vi "inteference V3.vi"(7 "number of points":i32, 8 "complex region":T1={"max re"=5.161869466666667e-06, "min re"=5.176843333333334e-06, "max im"=-2.467216e-05, "min im"=-0.001573233, "delta re"=0.003211203, "delta im"=0.00165815, "center re"=0.0015485608400000002, "delta  z"=0.0015530530000000002+0.0i, "center im"=0.0, "center z"=0.0+0.0i, "d im"=0.0, "d re"=0.0, "d z"=0.0+0.0i}, 9 "pond":cdb[][](array[numeric]), 10 "point sources":cdb[](array[numeric]), 11 "wave packet":cdb[][](array[numeric])) -> (3 "pond out":cdb[][](array[numeric]))   [LabVIEW 2010]
uses:
  complex region.ctl
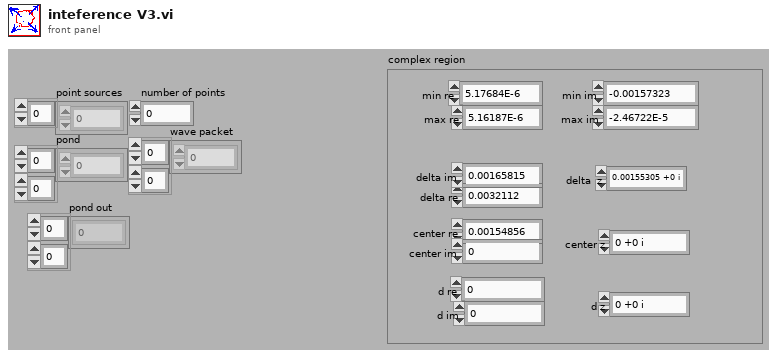
[diagram p1: front panel]
types:
  T1 = typedef "complex region.ctl" = cluster{"max re":dbl, "min re":dbl, "max im":dbl, "min im":dbl, "delta re":dbl, "delta im":dbl, "center re":dbl, "delta  z":cdb, "center im":dbl, "center z":cdb, "d im":dbl, "d re":dbl, "d z":cdb}
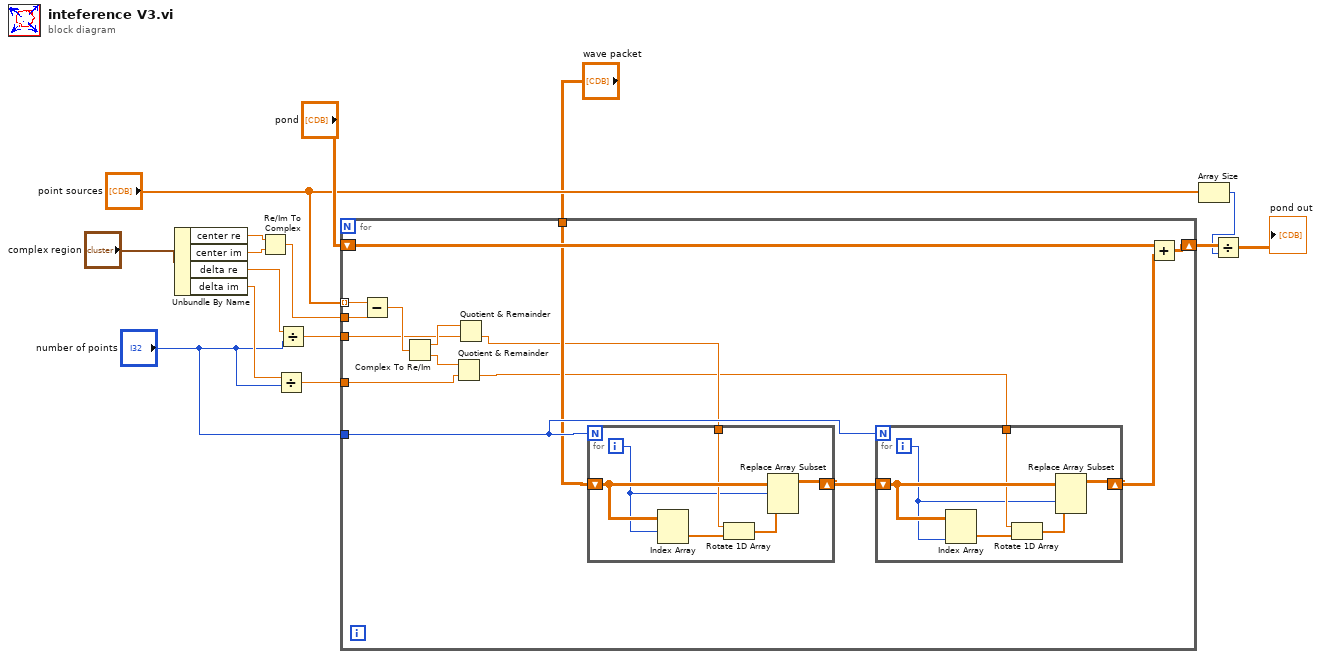
[diagram p0: block diagram]
diagram:
  n1 = Unbundle By Name("complex region") -> ("center re"=w15:dbl, "center im"=w14:dbl, "delta re"=w5:dbl, "delta im"=w4:dbl)
  n2 = Re/Im To Complex(1:w14, 2:w15) -> (0:w13:cdb)
  n3 = Divide(x=w4, y="number of points") -> (x/y=w2:dbl)
  n4 = Divide(x=w5, y="number of points") -> (x/y=w3:dbl)
  n5 = for {
    shift-right: [w29] -> w12
    shift-left: "pond" -> [w30]
    tunnel: "point sources" -> [w28] mode=indexing
    tunnel: "wave packet" -> [w18]
    tunnel: w13 -> [w27]
    tunnel: w3 -> [w24]
    tunnel: w2 -> [w22]
    tunnel: "number of points" -> [w20]
    n6 = Subtract(x=w28, y=w27) -> (x-y=w26:cdb)
    n7 = Complex To Re/Im(x + iy=w26) -> (x=w25:dbl, y=w23:dbl)
    n8 = Quotient & Remainder(x=w23, y=w22) -> (floor(x/y)=w16:dbl)  [unwired: 1 out]
    n9 = Quotient & Remainder(x=w25, y=w24) -> (floor(x/y)=w17:dbl)  [unwired: 1 out]
    n10 = for {
      N: w20 -> [_]
      shift-right: [w42] -> w21
      shift-left: w18 -> [w41]
      tunnel: w17 -> [w38]
      i -> [w37]
      n11 = Index Array(array=w41, index (row)=w37) -> (element=w39:cdb[])  [unwired: 1 in]
      n12 = Rotate 1D Array(1:w39, 2:w38) -> (0:w40:cdb[])
      n13 = Replace Array Subset(array=w41, new element=w40, index (row)=w37) -> (w42:cdb[][])  [unwired: 1 in]
    }
    n14 = for {
      N: w20 -> [_]
      shift-right: [w36] -> w19
      shift-left: w21 -> [w35]
      tunnel: w16 -> [w32]
      i -> [w31]
      n15 = Index Array(array=w35, index (col)=w31) -> (element=w33:cdb[])  [unwired: 1 in]
      n16 = Rotate 1D Array(1:w33, 2:w32) -> (0:w34:cdb[])
      n17 = Replace Array Subset(array=w35, new element=w34, index (col)=w31) -> (w36:cdb[][])  [unwired: 1 in]
    }
    n18 = Add(x=w30, y=w19) -> (x+y=w29:cdb[][])
  }
  n19 = Array Size(array="point sources") -> (size(s)=w11:i32)
  n20 = Divide(x=w12, y=w11) -> (x/y=→"pond out":cdb[][])
